vi "Drive Controller Interactive Check.vi"(8 "Interactive Command In":T1, 9 "Default Command":T1, 11 "Buttons":cluster{"Execute Cmd":bool, "Abort Cmd":bool}) -> (1 "Interactive Command Out":T1, 2 "Trace String":string, 3 "Schedule":bool)   [LabVIEW 2019]
doc: "Check the Execute and Abort buttons and choose the data and trace string."
uses:
  Drive Setpoints.ctl
  Drive Operations.ctl
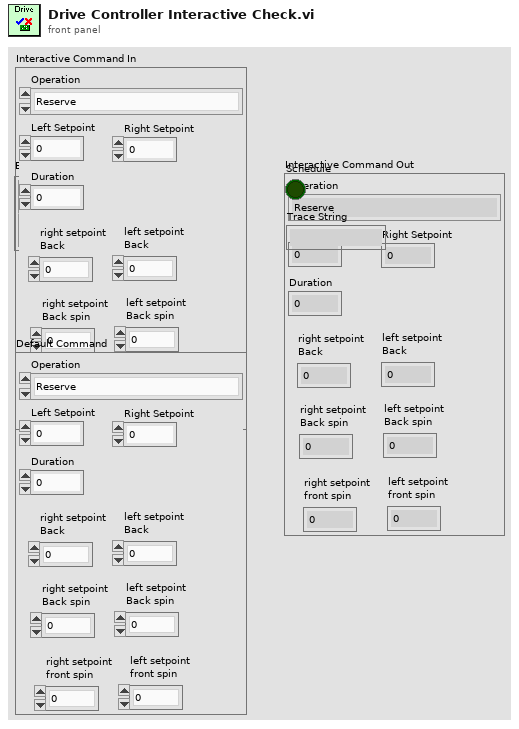
[diagram p1: front panel]
types:
  T1 = typedef "Drive Setpoints.ctl" = cluster{"Operation":T2, "Left Setpoint":dbl, "Right Setpoint":dbl, "Duration":dbl, "left setpoint\nBack":dbl, "right setpoint\nBack":dbl, "left setpoint\nBack spin":dbl, "right setpoint\nBack spin":dbl, "left setpoint \nfront spin":dbl, "right setpoint\nfront spin":dbl}
  T2 = typedef "Drive Operations.ctl" = enum16{"Reserve", "Read Current", "Immediate", "Drive for Time", "Drive for Distance"}
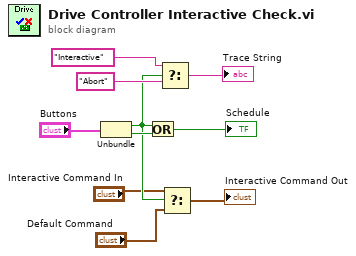
[diagram p0: block diagram]
diagram:
  n1 = Unbundle("Buttons") -> ("Execute Cmd"=w6:bool, "Abort Cmd"=w7:bool)
  n2 = Or(x=w6, y=w7) -> (x .or. y?=→"Schedule":bool)
  n3 = Select(t="Interactive", s=w6, f="Abort") -> (s? t:f=→"Trace String":string)
  n4 = Select(t="Interactive Command In", s=w6, f="Default Command") -> (s? t:f=→"Interactive Command Out":T1)
